vi "bit compare 1_0_x_lucid_test.vi"(9 "Input":bool[](array[boolean]), 10 "unsigned byte array":T1[](array[typedef])) -> (2 "x = y?":bool)   [LabVIEW 2020]
uses:
  byte.ctl
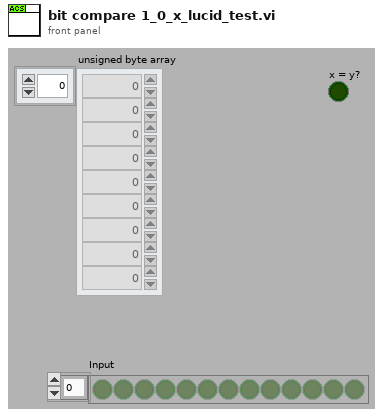
[diagram p1: front panel]
types:
  T1 = typedef "byte.ctl" = u8
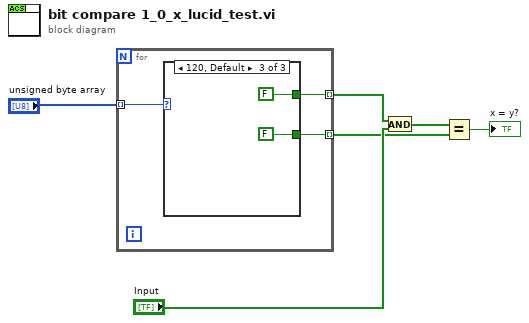
[diagram p0: block diagram]
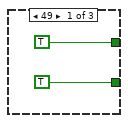
[diagram p2: hidden frame]
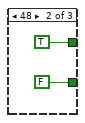
[diagram p3: hidden frame]
diagram:
  n1 = for {
    tunnel: "unsigned byte array" -> [w9] mode=indexing
    tunnel: [w8] -> w6 mode=indexing
    tunnel: [w7] -> w3 mode=indexing
    n2 = case shown="120, Default" w9 {
      tunnel: [TRUE TRUE FALSE] -> w8
      tunnel: [TRUE FALSE FALSE] -> w7
      frame 49 {
      }
      frame 48 {
      }
      frame 120, Default {
      }
    }
  }
  n3 = And(x=w6, y="Input") -> (x .and. y?=w4:bool[])
  n4 = Equal?(x=w4, y=w3) -> (x = y?=→"x = y?":bool)
